vi "resonant.raw queue to image queue_rrMD.vi"() -> ()   [LabVIEW 2012]
doc: "SciScan 1.2 160622"
uses:
  <vilib>/Utility/VariantDataType/Type.ctl
  GFG/GFGnumericGet.vi
  GFG/GFGbooleanGet.vi
  GFG/GFG library.lvlib
  <vilib>/Utility/VariantDataType/VariantType.lvlib
panel:
  out "Source VI":string
  out "size(s) 4":i32[](array[numeric])
  out "# elements in raw queue 2":i32
  out "error out 2":errorcluster
  out "error out 5":errorcluster
  out "size(s) 3":i32[](array[numeric])
  out "size(s) 2":i32[](array[numeric])
  out "size(s)":i32[](array[numeric])
  out "Numeric Control 2":i32
  out "Numeric Control":i32
  out "error out 4":errorcluster
  out "# elements in raw queue":i32
  out "error out":errorcluster
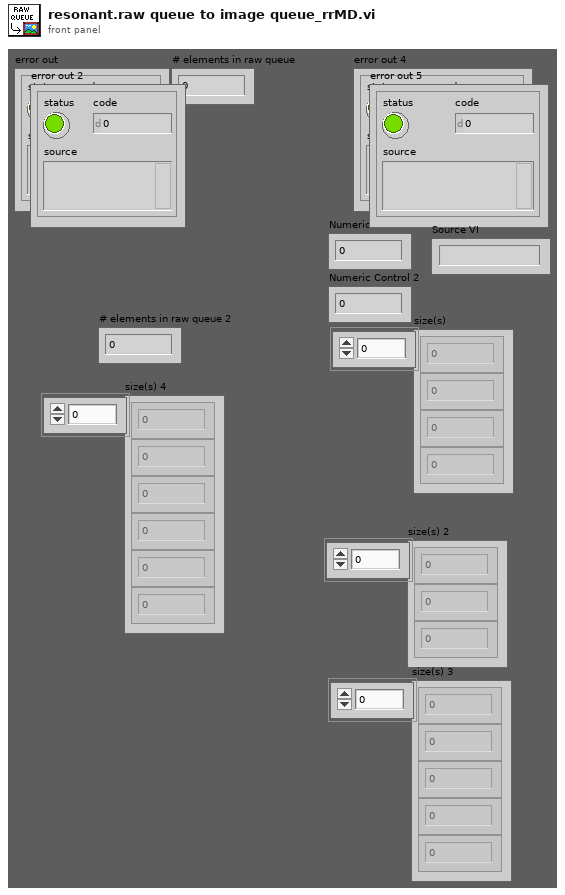
[diagram p1: front panel]
types:
  T1 = cluster{"NewVal":bool, "Event Registration Refnum":refnum<event-registration>}
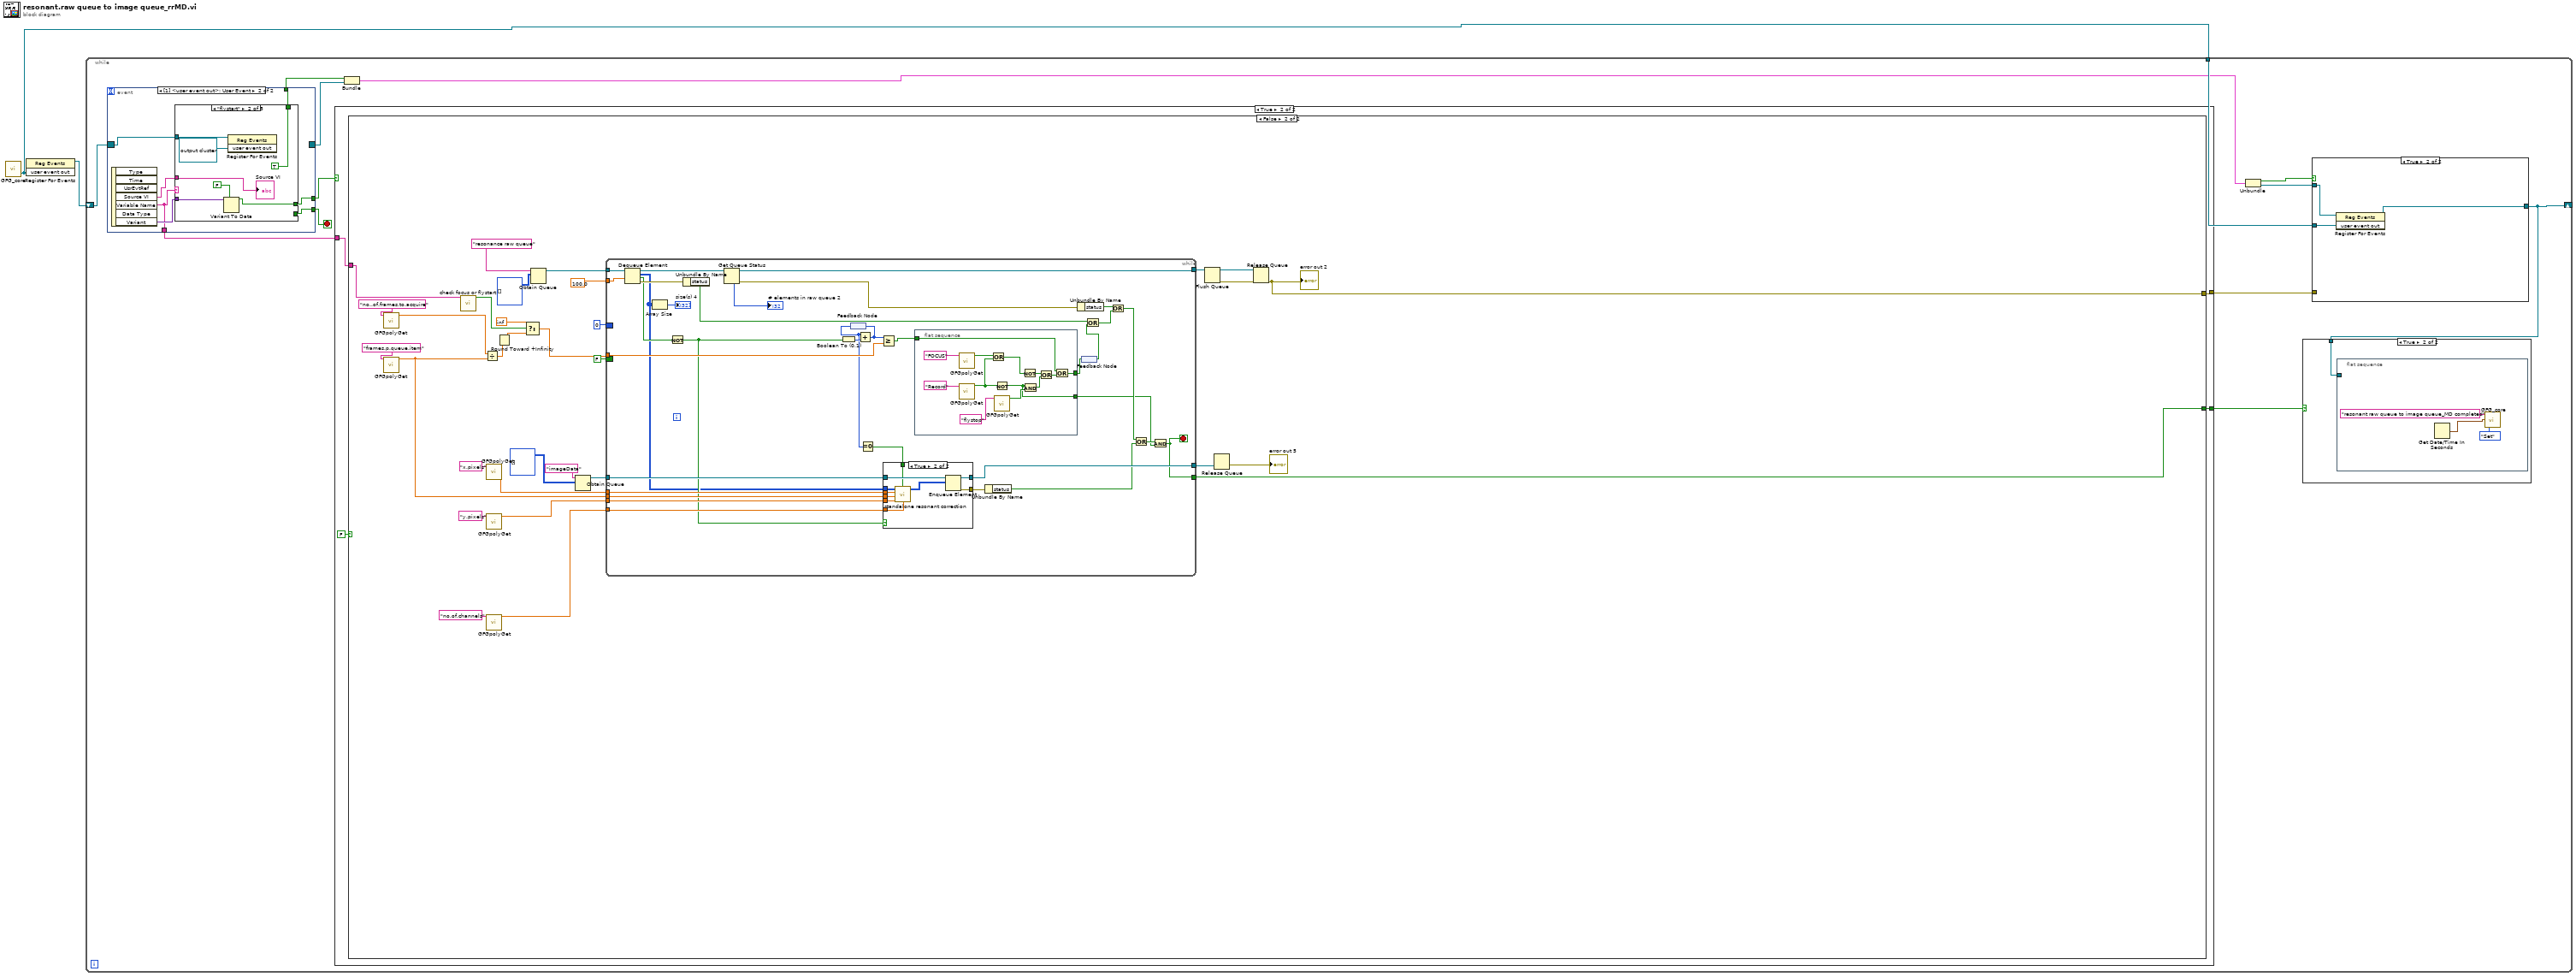
[diagram p0: block diagram]
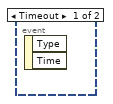
[diagram p4: hidden frame]
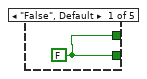
[diagram p5: hidden frame]
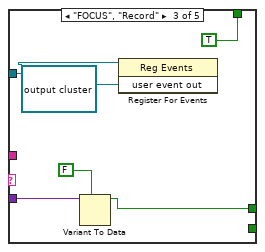
[diagram p6: hidden frame]
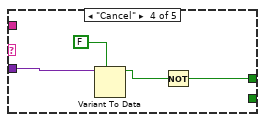
[diagram p7: hidden frame]
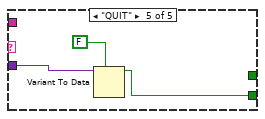
[diagram p8: hidden frame]
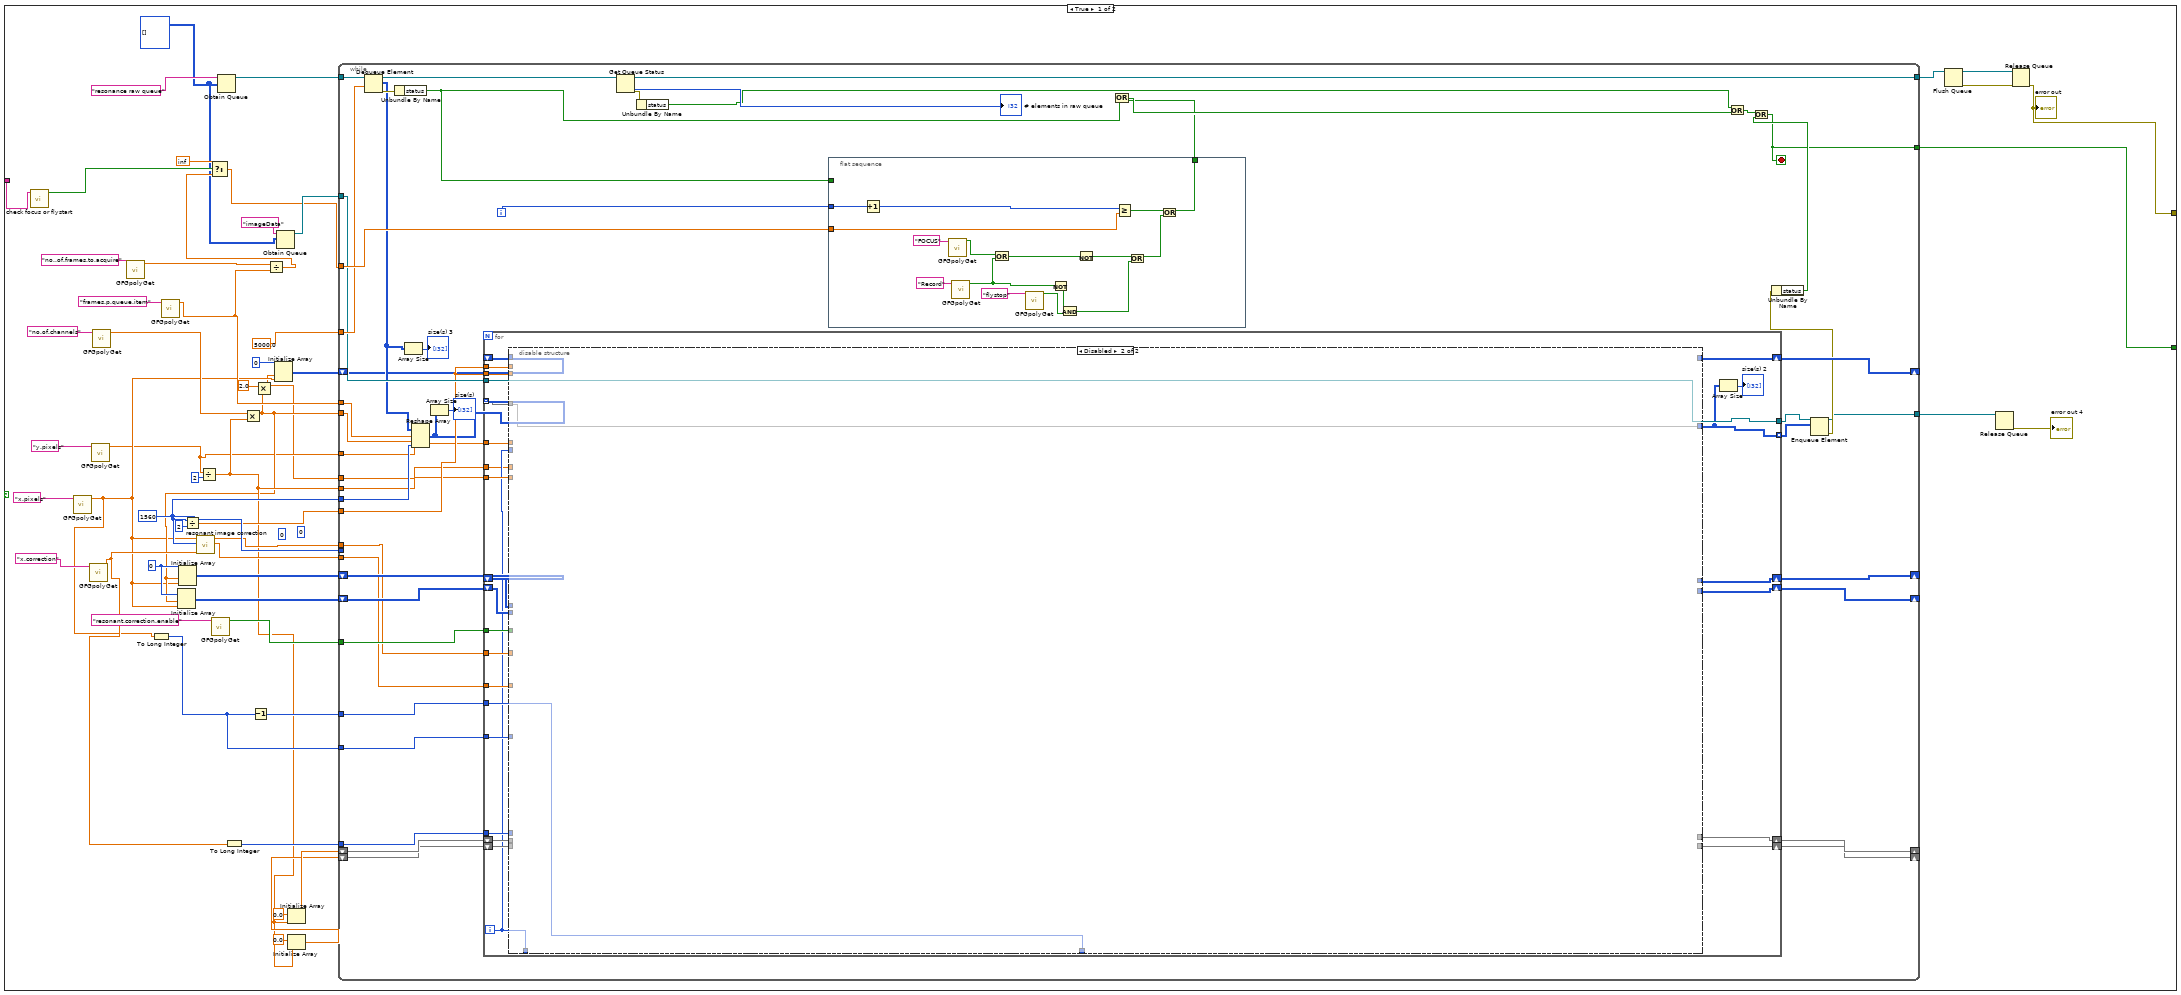
[diagram p10: hidden frame]
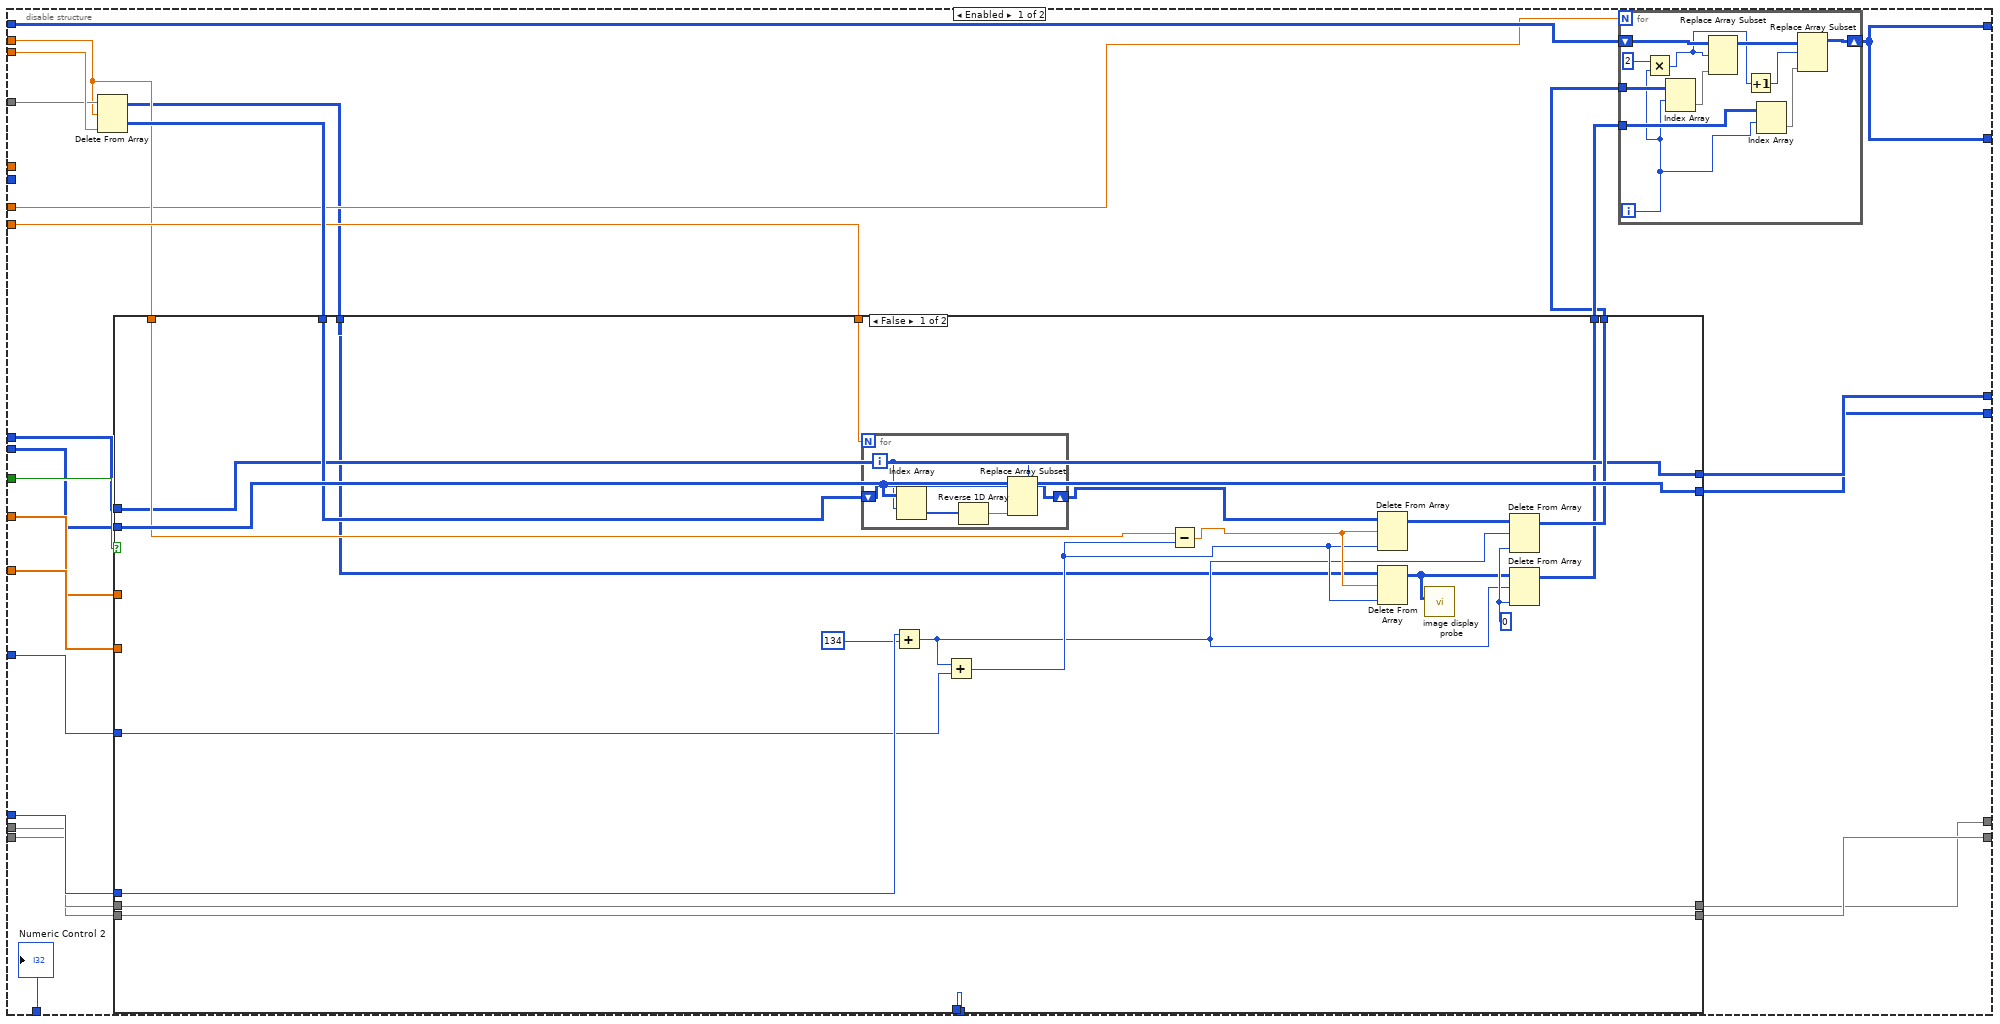
[diagram p11: hidden frame]
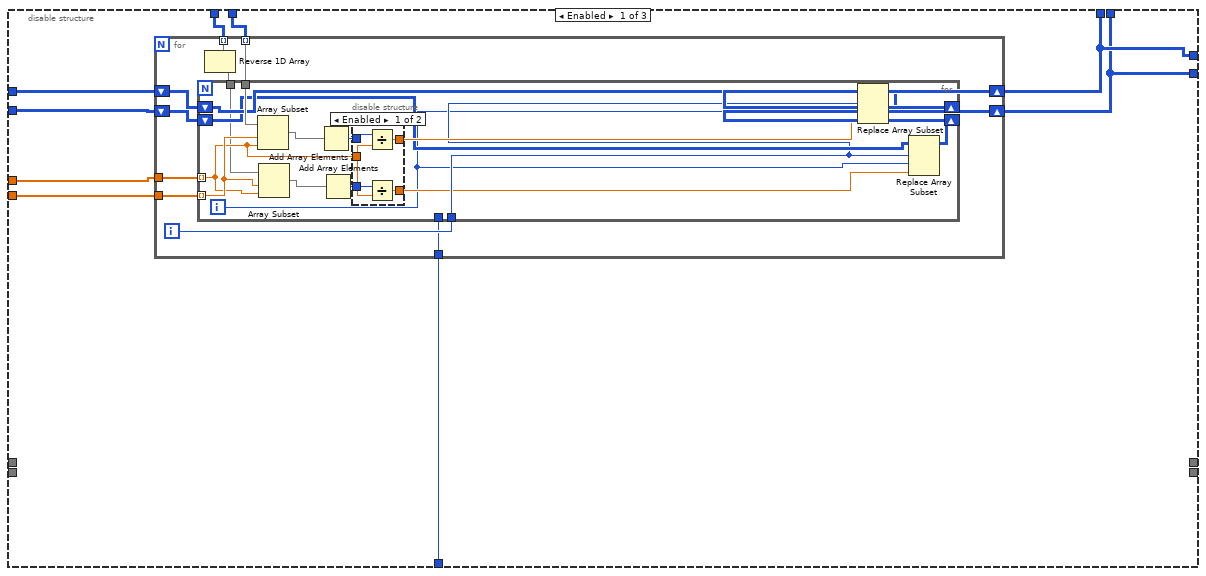
[diagram p13: hidden frame]
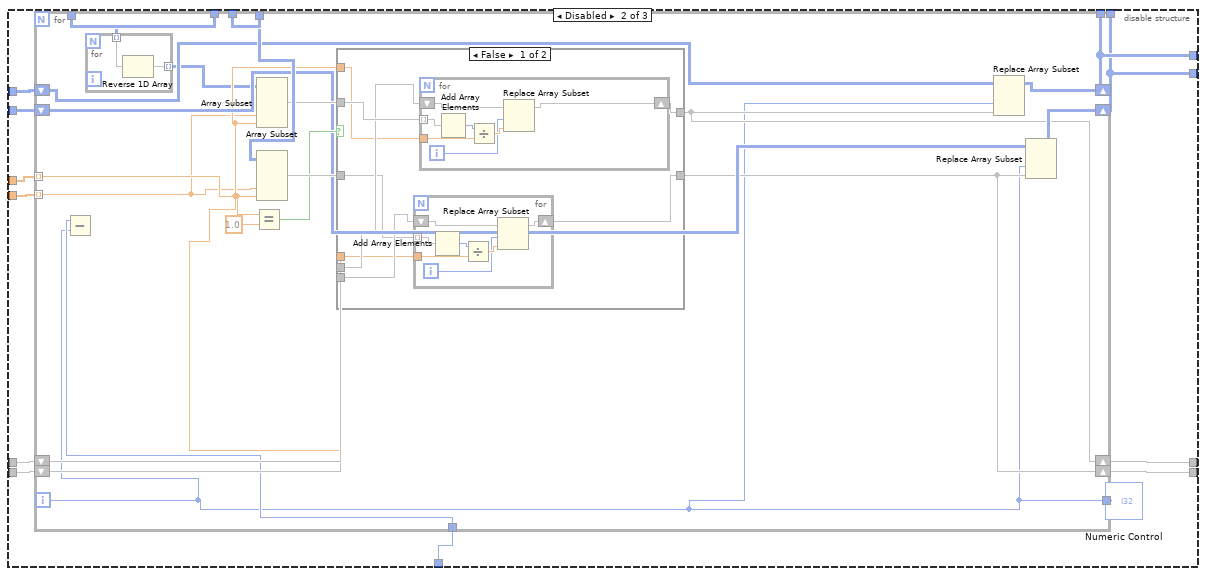
[diagram p15: hidden frame]
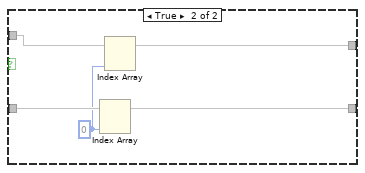
[diagram p16: hidden frame]
diagram:
  n1 = call "GFG_core.vi"() -> ("user event out"=w2:refnum<user-event>)  [unwired: 13 in, 6 out]
  n2 = register-events(w2) -> (reference out=w1:refnum<event-registration>)  [unwired: 2 in, 1 out]
  n3 = while {
    shift-right: [w3] -> _
    shift-left: w1 -> [w11]
    tunnel: w2 -> [w13]
    stop <- w14 stop-if-true
    n4 = event shown="[1] <user event out>: User Event" {
      selector: w11 -> [_ w27]
      dyn-events: [_ _] -> w9
      timeout: _ -> [_ _]
      tunnel: [_ w30] -> w15
      tunnel: [_ w29] -> w14
      tunnel: [_ w26] -> w10
      tunnel: [_ w25] -> w5
      event Timeout {
        n5 = event-data() -> ()  [unwired: 1 in, 2 out]
      }
      event User Event {
        n6 = event-data() -> ("Source VI"=w24:string, "Variable Name"=w25:string, "Variant"=w28:variant)  [unwired: 1 in, 4 out]
        n7 = case shown="\"flystart\"" w25 {
          tunnel: [w31 w36 w39 w45 _] -> w30
          tunnel: [w31 _ _ _ w49] -> w29
          tunnel: w28 -> [_ w37 w44 w47 w50]
          tunnel: w27 -> [_ w34 w41 _ _]
          tunnel: [_ TRUE ("NewVal") TRUE ("NewVal") _ _] -> w26
          tunnel: w24 -> [_ w32 _ _ _]
          frame "False", Default {
            w31 = FALSE ("NewVal")
          }
          frame "flystart" {
            n8 = Variant To Data(type=FALSE ("NewVal"), Variant=w37) -> (data=w36:bool)  [unwired: 1 in, 1 out]
            n9 = register-events(reference=w34, refnum<user-event> refnum ("user event out")) -> ()  [unwired: 1 in, 2 out]
            "Source VI" <- w32
          }
          frame "FOCUS", "Record" {
            n10 = Variant To Data(type=FALSE ("NewVal"), Variant=w44) -> (data=w39:bool)  [unwired: 1 in, 1 out]
            n11 = register-events(reference=w41, refnum<user-event> refnum ("user event out")) -> ()  [unwired: 1 in, 2 out]
          }
          frame "Cancel" {
            n12 = Variant To Data(type=FALSE ("NewVal"), Variant=w47) -> (data=w46:bool)  [unwired: 1 in, 1 out]
            n13 = Not(x=w46) -> (.not. x?=w45:bool)
          }
          frame "QUIT" {
            n14 = Variant To Data(type=FALSE ("NewVal"), Variant=w50) -> (data=w49:bool)  [unwired: 1 in, 1 out]
          }
        }
      }
    }
    n15 = case shown="True" w15 {
      tunnel: [_ w55] -> w12
      tunnel: w5 -> [_ w54]
      tunnel: [_ w53] -> w4
      frame False {
      }
      frame True {
        n16 = case shown="False" FALSE {
          tunnel: [w77 w399] -> w55
          tunnel: w54 -> [w73 w396]
          tunnel: [w71 w394] -> w53
          frame True {
            (unwired) u32 0
            (unwired) u32 0
            w92 = i16 0 ("sum")
            w86 = 1560 ("dimension size")
            w56 = i16[][][] [] ("initialized array")
            n17 = call "check focus or flystart.vi"("x"=w73) -> ("x .or. y?"=w72:bool)  [unwired: 10 in]
            n18 = call-poly "GFGpolyGet.vi"("Variable Name in"="x.pixels" ("Tag in")) -> ("Numeric"=w60:dbl)  [unwired: 8 in, 2 out]
            n19 = call-poly "GFGpolyGet.vi"("Variable Name in"="x.correction" ("Tag in")) -> ("Numeric"=w87:dbl)  [unwired: 8 in, 2 out]
            n20 = call-poly "GFGpolyGet.vi"("Variable Name in"="y.pixels" ("Tag in")) -> ("Numeric"=w58:dbl)  [unwired: 8 in, 2 out]
            n21 = call-poly "GFGpolyGet.vi"("Variable Name in"="no.of.channels" ("Tag in")) -> ("Numeric"=w69:dbl)  [unwired: 8 in, 2 out]
            n22 = call-poly "GFGpolyGet.vi"("Variable Name in"="no..of.frames.to.acquire" ("Tag in")) -> ("Numeric"=w101:dbl)  [unwired: 8 in, 2 out]
            n23 = To Long Integer(number=w60) -> (32bit integer=w68:i32)
            n24 = call-poly "GFGpolyGet.vi"("Variable Name in"="frames.p.queue.item" ("Tag in")) -> ("Numeric"=w65:dbl)  [unwired: 8 in, 2 out]
            n25 = Divide(x=w86, y=2) -> (x/y=w85:dbl)
            n26 = call "resonant image correction.vi"("shift index"=w87, "pixels per period (2pi, 2 lines)"=w86, "x pixels"=w60) -> ("histogram cumsum"=w79:dbl[], "histogram pixels to avg"=w78:dbl[])  [unwired: 7 in]
            n27 = Divide(x=w58, y=2) -> (x/y=w64:dbl)
            n28 = call-poly "GFGpolyGet.vi"("Variable Name in"="resonant.correction.enable" ("Tag in")) -> ("Boolean Value OUT"=w94:bool)  [unwired: 9 in, 1 out]
            n29 = Obtain Queue(name (unnamed)="resonance raw queue", element data type=w56) -> (queue out=w106:refnum<queue>)  [unwired: 3 in, 2 out]
            n30 = To Long Integer(number=w87) -> (32bit integer=w67:i32)
            n31 = Multiply(x=w69, y=w64) -> (x*y=w62:dbl)
            n32 = Initialize Array(w92, w62, w60) -> (w91:i16[][])
            n33 = Initialize Array(w92, w62, w60) -> (w90:i16[][])
            n34 = Decrement(x=w68) -> (x-1=w89:i32)
            n35 = Multiply(x=2.0, y=w62) -> (x*y=w57:dbl)
            n36 = Divide(x=w101, y=w65) -> (x/y=w75:dbl)
            n37 = Select(t=inf, s=w72, f=w75) -> (s? t:f=w74:dbl)
            n38 = Initialize Array(i16 0 ("sum"), w57, w60) -> (w59:i16[][])
            n39 = Obtain Queue(name (unnamed)="imageData", element data type=w56) -> (queue out=w107:refnum<queue>)  [unwired: 3 in, 2 out]
            n40 = Initialize Array(0.0 ("element"), w64) -> (w82:dbl[])
            n41 = Initialize Array(0.0 ("element"), w64) -> (w80:dbl[])
            n42 = while {
              tunnel: w106 -> [w152]
              tunnel: [w149] -> w105
              tunnel: w107 -> [w147]
              tunnel: w74 -> [w156]
              tunnel: 5000.0 -> [w153]
              tunnel: [w110] -> w98
              tunnel: w86 -> [w146]
              tunnel: w85 -> [w145]
              tunnel: w94 -> [w144]
              tunnel: w89 -> [w141]
              tunnel: w86 -> [_]
              tunnel: w79 -> [w136]
              tunnel: w78 -> [w135]
              tunnel: w67 -> [w134]
              shift-right: [w131] -> _
              shift-left: w82 -> [w133]
              shift-right: [w130] -> _
              shift-left: w80 -> [w132]
              shift-right: [w128] -> _
              shift-left: w91 -> [w143]
              shift-right: [w129] -> _
              shift-left: w90 -> [w142]
              tunnel: w68 -> [w127]
              tunnel: [w126] -> w71
              tunnel: w62 -> [w120]
              tunnel: w65 -> [w121]
              tunnel: w64 -> [w119]
              shift-right: [w117] -> _
              shift-left: w59 -> [w118]
              tunnel: w58 -> [w116]
              tunnel: w57 -> [w115]
              i -> [w154]
              stop <- w126 stop-if-true
              n43 = Dequeue Element(queue=w152, timeout in ms (-1)=w153) -> (queue out=w150:refnum<queue>, element=w123:i16[][][], error out=w155:errorcluster)  [unwired: 1 in, 1 out]
              n44 = Unbundle By Name(w155) -> ("status"=w125:bool)
              n45 = Array Size(array=w123) -> (size(s)=→"size(s) 3":i32[])
              n46 = Reshape Array(w123, w121, w120, w146) -> (w114:i16[][][])
              n47 = Array Size(array=w114) -> (size(s)=→"size(s)":i32[])
              n48 = for {
                tunnel: w114 -> [w183] mode=indexing
                tunnel: w145 -> [w199]
                tunnel: w145 -> [w198]
                tunnel: w147 -> [w175]
                tunnel: [w175] -> w112
                tunnel: w144 -> [w197]
                tunnel: w136 -> [w196]
                tunnel: w135 -> [w195]
                tunnel: w141 -> [w192]
                tunnel: [w174] -> w111 mode=indexing
                tunnel: w134 -> [w191]
                shift-right: [w187] -> w131
                shift-left: w133 -> [w190]
                shift-right: [w188] -> w130
                shift-left: w132 -> [w189]
                shift-right: [w186] -> w129
                shift-left: w142 -> [w193]
                shift-right: [w185] -> w128
                shift-left: w143 -> [w194]
                tunnel: w127 -> [w184]
                tunnel: w119 -> [w181]
                shift-right: [w179] -> w117
                shift-left: w118 -> [w180]
                tunnel: w116 -> [w177]
                tunnel: w115 -> [w176]
                i -> [w178]
                n49 = disable-structure shown="Disabled" {
                  disable-tunnel: w199 -> [w204 _]
                  disable-tunnel: w198 -> [w225 _]
                  disable-tunnel: w197 -> [w224 _]
                  disable-tunnel: w196 -> [w223 _]
                  disable-tunnel: w195 -> [w222 _]
                  disable-tunnel: w194 -> [w221 _]
                  disable-tunnel: w193 -> [w220 _]
                  disable-tunnel: [w202 w382] -> w174
                  disable-tunnel: w192 -> [w218 _]
                  disable-tunnel: w191 -> [w217 _]
                  disable-tunnel: w190 -> [w216 _]
                  disable-tunnel: w189 -> [w215 _]
                  disable-tunnel: [w214 _] -> w188
                  disable-tunnel: [w213 _] -> w187
                  disable-tunnel: [w212 _] -> w186
                  disable-tunnel: [w211 _] -> w185
                  disable-tunnel: w184 -> [w210 _]
                  disable-tunnel: w178 -> [w209 _]
                  disable-tunnel: w183 -> [w207 w382]
                  disable-tunnel: w181 -> [w208 _]
                  disable-tunnel: w180 -> [w205 _]
                  disable-tunnel: [w202 _] -> w179
                  disable-tunnel: w178 -> [_ _]
                  disable-tunnel: w177 -> [_ _]
                  disable-tunnel: w176 -> [w203 _]
                  frame Enabled {
                    n50 = Delete From Array(array=w207, length=w204, index (col)=w225) -> (deleted portion=w219:i16[][], array with subset deleted=w200:i16[][])  [unwired: 1 in]
                    n51 = case shown="False" w224 {
                      tunnel: w219 -> [w232 w265]
                      tunnel: w200 -> [w228 w264]
                      tunnel: w223 -> [_ w263]
                      tunnel: w222 -> [_ w262]
                      tunnel: w221 -> [w241 w261]
                      tunnel: w220 -> [w230 w260]
                      tunnel: [w227 w259] -> w206
                      tunnel: [w239 w258] -> w201
                      tunnel: w218 -> [_ w257]
                      tunnel: w217 -> [w244 _]
                      tunnel: w216 -> [w243 w256]
                      tunnel: [w243 w255] -> w213
                      tunnel: w215 -> [w242 w254]
                      tunnel: [w242 w253] -> w214
                      tunnel: [w230 w252] -> w212
                      tunnel: [w241 w251] -> w211
                      tunnel: w210 -> [w238 _]
                      tunnel: w208 -> [w233 _]
                      tunnel: w204 -> [w231 _]
                      frame False {
                        w245 = 0 ("disabled index (col)")
                        n52 = for {
                          N: w233 -> [_]
                          shift-right: [w249] -> w229
                          shift-left: w232 -> [w248]
                          i -> [w247]
                          n53 = Index Array(array=w248, index (row)=w247) -> (element=w246:i16[])  [unwired: 1 in]
                          n54 = Reverse 1D Array(array=w246) -> (reversed array=w250:i16[])
                          n55 = Replace Array Subset(array=w248, new element=w250, index (row)=w247) -> (w249:i16[][])  [unwired: 1 in]
                        }
                        n56 = Add(x=w244, y=134 ("length")) -> (x+y=w234:i32)
                        n57 = Add(x=w234, y=w238) -> (x+y=w235:i32)
                        n58 = Subtract(x=w231, y=w235) -> (x-y=w236:dbl)
                        n59 = Delete From Array(array=w229, length=w236, index (col)=w235) -> (array with subset deleted=w240:i16[][])  [unwired: 1 in, 1 out]
                        n60 = Delete From Array(array=w228, length=w236, index (col)=w235) -> (array with subset deleted=w226:i16[][])  [unwired: 1 in, 1 out]
                        n61 = call "image display probe.vi"("Image Pixels (I16)"=w226) -> ()  [unwired: 11 in]
                        n62 = Delete From Array(array=w240, length=w234, index (col)=w245) -> (array with subset deleted=w239:i16[][])  [unwired: 1 in, 1 out]
                        n63 = Delete From Array(array=w226, length=w234, index (col)=w245) -> (array with subset deleted=w227:i16[][])  [unwired: 1 in, 1 out]
                      }
                      frame True {
                        n64 = disable-structure shown="Disabled" {
                          disable-tunnel: w265 -> [w274 w322 _]
                          disable-tunnel: w264 -> [w273 w321 _]
                          disable-tunnel: w263 -> [w272 w320 _]
                          disable-tunnel: w262 -> [w271 w309 _]
                          disable-tunnel: w261 -> [w270 w319 _]
                          disable-tunnel: w260 -> [w269 w318 _]
                          disable-tunnel: [w267 w312 _] -> w259
                          disable-tunnel: [w266 w311 _] -> w258
                          disable-tunnel: w257 -> [w268 w317 _]
                          disable-tunnel: w256 -> [_ w316 _]
                          disable-tunnel: [_ w315 _] -> w255
                          disable-tunnel: w254 -> [_ w314 _]
                          disable-tunnel: [_ w313 _] -> w253
                          disable-tunnel: [w267 w312 _] -> w252
                          disable-tunnel: [w266 w311 _] -> w251
                          frame Enabled {
                            n65 = for {
                              tunnel: w274 -> [w283] mode=indexing
                              tunnel: w273 -> [w282] mode=indexing
                              tunnel: w272 -> [w285]
                              tunnel: w271 -> [w284]
                              shift-right: [w277] -> w266
                              shift-left: w270 -> [w281]
                              shift-right: [w278] -> w267
                              shift-left: w269 -> [w280]
                              tunnel: w268 -> [w276]
                              i -> [w279]
                              n66 = Reverse 1D Array(array=w283) -> (reversed array=w275:i16[])
                              n67 = for {
                                tunnel: w285 -> [w300] mode=indexing
                                tunnel: w284 -> [w295] mode=indexing
                                tunnel: w275 -> [w286]
                                tunnel: w282 -> [w301]
                                shift-right: [w288] -> w277
                                shift-left: w281 -> [w292]
                                shift-right: [w289] -> w278
                                shift-left: w280 -> [w293]
                                tunnel: w279 -> [w291]
                                tunnel: w276 -> [_]
                                i -> [w287]
                                n68 = Array Subset(array=w301, index=w300, length=w295) -> (w299:i16[])
                                n69 = Array Subset(array=w286, index=w300, length=w295) -> (w298:i16[])
                                n70 = Add Array Elements(numeric array=w299) -> (sum=w297:i16)
                                n71 = Add Array Elements(numeric array=w298) -> (sum=w296:i16)
                                n72 = disable-structure shown="Enabled" {
                                disable-tunnel: w297 -> [w306 w308]
                                disable-tunnel: w296 -> [w305 w307]
                                disable-tunnel: w295 -> [w304 _]
                                disable-tunnel: [w303 w308] -> w294
                                disable-tunnel: [w302 w307] -> w290
                                frame Enabled {
                                n73 = Divide(x=w306, y=w304) -> (x/y=w303:dbl)
                                n74 = Divide(x=w305, y=w304) -> (x/y=w302:dbl)
                                }
                                frame Disabled {
                                }
                                }
                                n75 = Replace Array Subset(array=w293, new element=w294, index (row)=w291, index (col)=w287) -> (w289:i16[][])
                                n76 = Replace Array Subset(array=w292, new element=w290, index (row)=w291, index (col)=w287) -> (w288:i16[][])
                              }
                            }
                          }
                          frame Disabled {
                            n77 = for {
                              tunnel: w322 -> [w324]
                              tunnel: w321 -> [w341]
                              tunnel: w320 -> [w325] mode=indexing
                              tunnel: w309 -> [w326] mode=indexing
                              shift-right: [w335] -> w311
                              shift-left: w319 -> [w334]
                              shift-right: [w336] -> w312
                              shift-left: w318 -> [w333]
                              tunnel: w317 -> [w328]
                              shift-right: [w330] -> w315
                              shift-left: w316 -> [w332]
                              shift-right: [w329] -> w313
                              shift-left: w314 -> [w331]
                              tunnel: [w327] -> w310
                              i -> [w327]
                              n78 = Subtract(x=w328, y=w327) -> ()  [unwired: 1 out]
                              n79 = for {
                                tunnel: w324 -> [w343] mode=indexing
                                tunnel: [w342] -> w323 mode=indexing
                                n80 = Reverse 1D Array(array=w343) -> (reversed array=w342:i16[])
                              }
                              n81 = Equal?(x=w326, y=1.0) -> (x = y?=w337:bool)
                              n82 = Array Subset(array=w323, index (col)=w325, length (col)=w326) -> (w339:i16[][])  [unwired: 2 in]
                              n83 = Array Subset(array=w341, index (col)=w325, length (col)=w326) -> (w340:i16[][])  [unwired: 2 in]
                              n84 = case shown="False" w337 {
                                tunnel: w340 -> [w347 w369]
                                tunnel: w339 -> [w351 w370]
                                tunnel: [w349 w368] -> w330
                                tunnel: [w345 w367] -> w329
                                tunnel: w326 -> [w346 _]
                                tunnel: w332 -> [w350 _]
                                tunnel: w331 -> [w348 _]
                                tunnel: w326 -> [w344 _]
                                frame False {
                                n85 = for {
                                tunnel: w347 -> [w358] mode=indexing
                                shift-right: [w352] -> w345
                                shift-left: w348 -> [w355]
                                tunnel: w344 -> [w356]
                                i -> [w353]
                                n86 = Add Array Elements(numeric array=w358) -> (sum=w357:i16)
                                n87 = Divide(x=w357, y=w356) -> (x/y=w354:dbl)
                                n88 = Replace Array Subset(array=w355, new element=w354, index=w353) -> (w352:dbl[])
                                }
                                n89 = for {
                                tunnel: w351 -> [w365] mode=indexing
                                shift-right: [w360] -> w349
                                shift-left: w350 -> [w362]
                                tunnel: w346 -> [w363]
                                i -> [w359]
                                n90 = Add Array Elements(numeric array=w365) -> (sum=w364:i16)
                                n91 = Divide(x=w364, y=w363) -> (x/y=w361:dbl)
                                n92 = Replace Array Subset(array=w362, new element=w361, index=w359) -> (w360:dbl[])
                                }
                                }
                                frame True {
                                w366 = 0 ("disabled index (col)")
                                n93 = Index Array(array=w369, index (col)=w366) -> (element=w367:i16[])  [unwired: 1 in]
                                n94 = Index Array(array=w370, index (col)=w366) -> (element=w368:i16[])  [unwired: 1 in]
                                }
                              }
                              n95 = Replace Array Subset(array=w333, new element=w330, index (col)=w327) -> (w336:i16[][])  [unwired: 1 in]
                              n96 = Replace Array Subset(array=w334, new element=w329, index (col)=w327) -> (w335:i16[][])  [unwired: 1 in]
                            }
                            "Numeric Control" <- w310
                          }
                          frame Disabled {
                          }
                        }
                      }
                    }
                    n97 = for {
                      N: w203 -> [_]
                      shift-right: [w377] -> w202
                      shift-left: w205 -> [w379]
                      tunnel: w201 -> [w381]
                      tunnel: w206 -> [w380]
                      i -> [w372]
                      n98 = Multiply(x=2, y=w372) -> (x*y=w371:i32)
                      n99 = Index Array(array=w381, index (row)=w372) -> (element=w376:i16[])  [unwired: 1 in]
                      n100 = Replace Array Subset(array=w379, new element=w376, index (row)=w371) -> (w378:i16[][])  [unwired: 1 in]
                      n101 = Increment(x=w371) -> (x+1=w373:i32)
                      n102 = Index Array(array=w380, index (row)=w372) -> (element=w375:i16[])  [unwired: 1 in]
                      n103 = Replace Array Subset(array=w378, new element=w375, index (row)=w373) -> (w377:i16[][])  [unwired: 1 in]
                    }
                    "Numeric Control 2" <- w209
                  }
                  frame Disabled {
                  }
                }
                n104 = Array Size(array=w174) -> (size(s)=→"size(s) 2":i32[])
              }
              n105 = Get Queue Status(queue=w150) -> (queue out=w149:refnum<queue>, error out=w139:errorcluster, # elements in queue=→"# elements in raw queue":i32)  [unwired: 2 in, 5 out]
              n106 = Unbundle By Name(w139) -> ("status"=w138:bool)
              n107 = flat-sequence {
                tunnel: w156 -> [w173]
                tunnel: w154 -> [w171]
                tunnel: [w167] -> w151
                tunnel: w125 -> [_]
                frame #0 {
                  n108 = Increment(x=w171) -> (x+1=w165:i32)
                  n109 = call-poly "GFGpolyGet.vi"("Variable Name in"="FOCUS") -> ("Boolean Value OUT"=w168:bool)  [unwired: 9 in, 1 out]
                  n110 = call-poly "GFGpolyGet.vi"("Variable Name in"="Record") -> ("Boolean Value OUT"=w160:bool)  [unwired: 9 in, 1 out]
                  n111 = Or(x=w168, y=w160) -> (x .or. y?=w166:bool)
                  n112 = call-poly "GFGpolyGet.vi"("Variable Name in"="flystop") -> ("Boolean Value OUT"=w161:bool)  [unwired: 9 in, 1 out]
                  n113 = Not(x=w160) -> (.not. x?=w162:bool)
                  n114 = And(x=w162, y=w161) -> (x .and. y?=w158:bool)
                  n115 = Not(x=w166) -> (.not. x?=w164:bool)
                  n116 = Greater Or Equal?(x=w165, y=w173) -> (x >= y?=w172:bool)
                  n117 = Or(x=w164, y=w158) -> (x .or. y?=w159:bool)
                  n118 = Or(x=w172, y=w159) -> (x .or. y?=w167:bool)
                }
              }
              n119 = Or(x=w125, y=w151) -> (x .or. y?=w157:bool)
              n120 = Or(x=w138, y=w157) -> (x .or. y?=w140:bool)
              n121 = Enqueue Element(queue=w112, element=w111) -> (queue out=w110:refnum<queue>, error out=w113:errorcluster)  [unwired: 2 in, 1 out]
              n122 = Unbundle By Name(w113) -> ("status"=w137:bool)
              n123 = Or(x=w140, y=w137) -> (x .or. y?=w126:bool)
            }
            n124 = Flush Queue(queue=w105) -> (queue out=w104:refnum<queue>, error out=w100:errorcluster)  [unwired: 1 in, 1 out]
            n125 = Release Queue(queue=w98) -> (error out=→"error out 4":errorcluster)  [unwired: 2 in, 2 out]
            n126 = Release Queue(queue=w104, error in (no error)=w100) -> (error out=w77:errorcluster)  [unwired: 1 in, 2 out]
            "error out" <- w77
          }
          frame False {
            n127 = call-poly "GFGpolyGet.vi"("Variable Name in"="no..of.frames.to.acquire" ("Tag in")) -> ("Numeric"=w406:dbl)  [unwired: 8 in, 2 out]
            n128 = call-poly "GFGpolyGet.vi"("Variable Name in"="frames.p.queue.item" ("Tag in")) -> ("Numeric"=w390:dbl)  [unwired: 8 in, 2 out]
            n129 = call "check focus or flystart.vi"("x"=w396) -> ("x .or. y?"=w395:bool)  [unwired: 10 in]
            n130 = Divide(x=w406, y=w390) -> (x/y=w385:dbl)
            n131 = call-poly "GFGpolyGet.vi"("Variable Name in"="x.pixels" ("Tag in")) -> ("Numeric"=w389:dbl)  [unwired: 8 in, 2 out]
            n132 = call-poly "GFGpolyGet.vi"("Variable Name in"="y.pixels" ("Tag in")) -> ("Numeric"=w391:dbl)  [unwired: 8 in, 2 out]
            n133 = call-poly "GFGpolyGet.vi"("Variable Name in"="no.of.channels" ("Tag in")) -> ("Numeric"=w388:dbl)  [unwired: 8 in, 2 out]
            n134 = Round Toward +Infinity(x=w385) -> (ceil(x): smallest int >= x=w386:dbl)
            n135 = Select(t=inf, s=w395, f=w386) -> (s? t:f=w397:dbl)
            n136 = Obtain Queue(name (unnamed)="resonance raw queue", element data type=i16[][][] [] ("initialized array")) -> (queue out=w411:refnum<queue>)  [unwired: 3 in, 2 out]
            n137 = Obtain Queue(name (unnamed)="imageData", element data type=i16[][][] [] ("initialized array")) -> (queue out=w412:refnum<queue>)  [unwired: 3 in, 2 out]
            n138 = while {
              tunnel: w411 -> [w445]
              tunnel: [w442] -> w410
              tunnel: w412 -> [w441]
              tunnel: w397 -> [w426]
              tunnel: 100.0 -> [w446]
              tunnel: [w440] -> w402
              tunnel: [w418] -> w394
              tunnel: w391 -> [w433]
              tunnel: w390 -> [w432]
              tunnel: w389 -> [w431]
              tunnel: w388 -> [w430]
              border: i16 0 -> [_]
              border: FALSE -> [_]
              stop <- w418 stop-if-true
              n139 = Dequeue Element(queue=w445, timeout in ms (-1)=w446) -> (queue out=w443:refnum<queue>, element=w420:i16[][][], timed out?=w428:bool, error out=w447:errorcluster)  [unwired: 1 in]
              n140 = Array Size(array=w420) -> (size(s)=→"size(s) 4":i32[])
              n141 = Not(x=w428) -> (.not. x?=w424:bool)
              n142 = Unbundle By Name(w447) -> ("status"=w434:bool)
              n143 = Get Queue Status(queue=w443) -> (queue out=w442:refnum<queue>, error out=w438:errorcluster, # elements in queue=→"# elements in raw queue 2":i32)  [unwired: 2 in, 5 out]
              n144 = Boolean To (0,1)(Boolean=w424) -> (0, 1=w427:i16)
              n145 = feedback #1() -> (w422:i16)
              n146 = Add(x=w422, y=w427) -> (x+y=w423:i16)
              n147 = feedback-in #1(w423) -> ()
              n148 = Equal To 0?(x=w422) -> (x = 0?=w421:bool)
              n149 = Greater Or Equal?(x=w423, y=w426) -> (x >= y?=w425:bool)
              n150 = case shown="True" w424 {
                tunnel: w441 -> [w449 w459]
                tunnel: [w449 w458] -> w440
                tunnel: [_ w457] -> w436
                tunnel: w433 -> [_ w456]
                tunnel: w432 -> [_ w455]
                tunnel: w431 -> [_ w454]
                tunnel: w430 -> [_ w453]
                tunnel: w420 -> [_ w451]
                tunnel: w421 -> [_ w450]
                frame False {
                }
                frame True {
                  n151 = call "standalone resonant correction.vi"("uncorrected images in"=w451, "force reset shift registers"=w450, "frames.p.queue.item"=w455, "x.pixels"=w454, "y.pixels"=w456, "no.of.channels"=w453) -> ("corrected images out"=w452:i16[][][])  [unwired: 9 in]
                  n152 = Enqueue Element(queue=w459, element=w452) -> (queue out=w458:refnum<queue>, error out=w457:errorcluster)  [unwired: 2 in, 1 out]
                }
              }
              n153 = flat-sequence {
                tunnel: [w469] -> w444
                tunnel: w425 -> [w461]
                tunnel: [w460] -> w416
                frame #0 {
                  n154 = call-poly "GFGpolyGet.vi"("Variable Name in"="FOCUS") -> ("Boolean Value OUT"=w470:bool)  [unwired: 9 in, 1 out]
                  n155 = call-poly "GFGpolyGet.vi"("Variable Name in"="Record") -> ("Boolean Value OUT"=w464:bool)  [unwired: 9 in, 1 out]
                  n156 = Or(x=w470, y=w464) -> (x .or. y?=w468:bool)
                  n157 = Not(x=w464) -> (.not. x?=w460:bool)
                  n158 = call-poly "GFGpolyGet.vi"("Variable Name in"="flystop") -> ("Boolean Value OUT"=w465:bool)  [unwired: 9 in, 1 out]
                  n159 = Not(x=w468) -> (.not. x?=w467:bool)
                  n160 = And(x=w460, y=w465) -> (x .and. y?=w462:bool)
                  n161 = Or(x=w467, y=w462) -> (x .or. y?=w463:bool)
                  n162 = Or(x=w461, y=w463) -> (x .or. y?=w469:bool)
                }
              }
              n163 = Unbundle By Name(w436) -> ("status"=w435:bool)
              n164 = Unbundle By Name(w438) -> ("status"=w437:bool)
              n165 = feedback-in #2(w444) -> ()
              n166 = feedback #2() -> (w415:bool)
              n167 = Or(x=w434, y=w415) -> (x .or. y?=w448:bool)
              n168 = Or(x=w437, y=w448) -> (x .or. y?=w439:bool)
              n169 = Or(x=w439, y=w435) -> (x .or. y?=w419:bool)
              n170 = And(x=w419, y=w416) -> (x .and. y?=w418:bool)
            }
            n171 = Flush Queue(queue=w410) -> (queue out=w409:refnum<queue>, error out=w405:errorcluster)  [unwired: 1 in, 1 out]
            n172 = Release Queue(queue=w402) -> (error out=→"error out 5":errorcluster)  [unwired: 2 in, 2 out]
            n173 = Release Queue(queue=w409, error in (no error)=w405) -> (error out=w399:errorcluster)  [unwired: 1 in, 2 out]
            "error out 2" <- w399
          }
        }
      }
    }
    n174 = Bundle("NewVal"=w10, "Event Registration Refnum"=w9) -> (w8:T1)  [unwired: 1 in]
    n175 = Unbundle(w8) -> ("NewVal"=w7:bool, "Event Registration Refnum"=w6:refnum<event-registration>)
    n176 = case shown="True" w7 {
      tunnel: [w20 w23] -> w3
      tunnel: w13 -> [_ w22]
      tunnel: w12 -> [_ _]
      tunnel: w6 -> [w20 w21]
      frame False {
      }
      frame True {
        n177 = register-events(reference=w21, w22) -> (reference out=w23:refnum<event-registration>)  [unwired: 1 in, 1 out]
      }
    }
    n178 = case shown="True" w4 {
      tunnel: w3 -> [_ w16]
      frame False {
      }
      frame True {
        n179 = flat-sequence {
          tunnel: w16 -> [_]
          frame #0 {
            n180 = Get Date/Time In Seconds() -> (seconds since 1Jan1904=w17:timestamp)
            n181 = call "GFG_core.vi"("Variable Name in"="resonant raw queue to image queue_MD completed", "Variant in"=w17, "Action"=enum16{"Init", "Set", "Get"}."Set") -> ()  [unwired: 10 in, 7 out]
          }
        }
      }
    }
  }
